vi "Init TCP.vi"(8 "error in (no error)":errorcluster, 11 "Vecto in":refnum<class "Vecto.lvclass">) -> (0 "error out":errorcluster, 3 "Vecto out":refnum<class "Vecto.lvclass">)   [LabVIEW 2020, in "Vecto.lvlib" / "Vecto.lvclass"]
uses:
  Vecto.lvclass
  Node Config/Node Config.lvclass
  TCPMessaging/TCPMessaging.lvclass
  VectoTCPConnectionHandler/VectoTCPConnectionHandler.lvclass
  proto/TcpClientHello/Data.ctl
  proto/TcpClientHello/TcpClientHello.lvlib
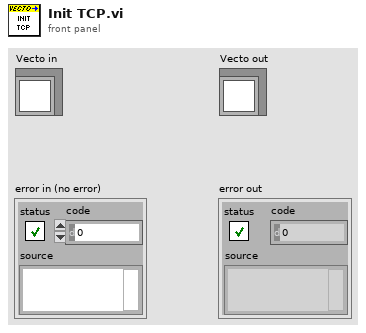
[diagram p1: front panel]
types:
  T1 = typedef "TcpClientHello.lvlib/Data.ctl" = cluster{"node_id":u32, "system":string, "cluster":string, "node_name":string, "app_version":string, "config_version":string}
  T2 = typedef "Vecto.lvlib/Node Config.lvclass/Node Info.ctl" = cluster{"System":string, "Cluster":string, "Name":string, "ID":u32}
  T3 = typedef "Vecto.lvlib/Node Config.lvclass/TCP Messaging Info.ctl" = cluster{"Address":string, "Port":u16, "Server (Client)":bool}
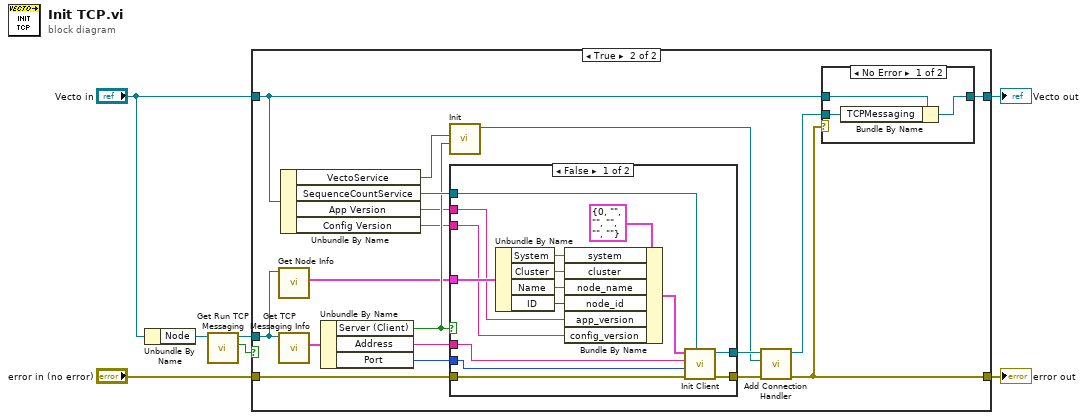
[diagram p0: block diagram]
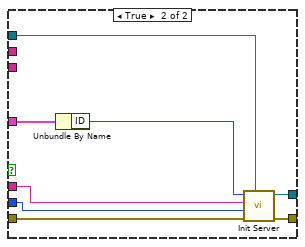
[diagram p3: hidden frame]
diagram:
  n1 = Unbundle By Name("Vecto in") -> ("Node"=w7:refnum<class "Node Config.lvclass">)
  n2 = call "Get Run TCP Messaging.vi"("Node Config in"=w7) -> ("Run TCP Messaging"=w6:bool, "Node Config out"=w4:refnum<class "Node Config.lvclass">)  [unwired: 8 in, 1 out]
  n3 = case shown="True" w6 {
    tunnel: "error in (no error)" -> [w8 w27]
    tunnel: w4 -> [_ w13]
    tunnel: "Vecto in" -> [w9 w22]
    tunnel: [w8 w17] -> w2
    tunnel: [w9 w21] -> w1
    frame False {
    }
    frame True {
      n4 = call "Get Node Info.vi"("Node Config in"=w13) -> ("Info"=w12:T2)  [unwired: 8 in, 2 out]
      n5 = call "Get TCP Messaging Info.vi"("Node Config in"=w13) -> ("TCP Messaging Info"=w26:T3)  [unwired: 8 in, 2 out]
      n6 = Unbundle By Name(w22) -> ("VectoService"=w19:refnum<class "VectoInfo.lvclass">, "SequenceCountService"=w23:refnum<class "SequenceCountService.lvclass">, "App Version"=w10:string, "Config Version"=w11:string)
      n7 = Unbundle By Name(w26) -> ("Server (Client)"=w18:bool, "Address"=w25:string, "Port"=w24:u16)
      n8 = call "Init.vi"("Server (Client)"=w18, "VectoInfo"=w19) -> ("VectoTCPConnectionHandler out"=w14:refnum<class "VectoTCPConnectionHandler.lvclass">)  [unwired: 8 in, 1 out]
      n9 = case shown="False" w18 {
        tunnel: w27 -> [w42 w50]
        tunnel: w25 -> [w32 w49]
        tunnel: w24 -> [w31 w48]
        tunnel: w23 -> [w39 w47]
        tunnel: [w40 w46] -> w16
        tunnel: [w41 w45] -> w20
        tunnel: w12 -> [w36 w44]
        tunnel: w11 -> [w30 _]
        tunnel: w10 -> [w29 _]
        frame False {
          n10 = Unbundle By Name(w36) -> ("System"=w35:string, "Cluster"=w34:string, "Name"=w33:string, "ID"=w28:u32)
          n11 = Bundle By Name(cluster=T1 {"node_id"=0, "system"="", "cluster"="", "node_name"="", "app_version"="", "config_version"=""} ("Client Info"), "system"=w35, "cluster"=w34, "node_name"=w33, "node_id"=w28, "app_version"=w29, "config_version"=w30) -> (w37:T1)
          n12 = call "Init Client.vi"("SequenceCountService"=w39, "error in (no error)"=w42, "Remote Port"=w31, "Remote Address"=w32, "Client Info"=w37) -> ("error out"=w41:errorcluster, "TCPMessaging out"=w40:refnum<class "TCPMessaging.lvclass">)  [unwired: 5 in]
        }
        frame True {
          n13 = Unbundle By Name(w44) -> ("ID"=w43:u32)
          n14 = call "Init Server.vi"("SequenceCountService"=w47, "error in (no error)"=w50, "Bind Port"=w48, "Bind Address"=w49, "Node ID"=w43) -> ("error out"=w45:errorcluster, "TCPMessaging out"=w46:refnum<class "TCPMessaging.lvclass">)  [unwired: 5 in]
        }
      }
      n15 = call "Add Connection Handler.vi"("error in (no error)"=w20, "TCPConnectionHandler"=w14, "TCPMessaging in"=w16) -> ("error out"=w17:errorcluster, "TCPMessaging out"=w15:refnum<class "TCPMessaging.lvclass">)  [unwired: 7 in]
      n16 = case shown="No Error" w17 {
        tunnel: w22 -> [w53 w54]
        tunnel: w15 -> [w52 _]
        tunnel: [w51 w54] -> w21
        frame No Error {
          n17 = Bundle By Name(cluster=w53, "TCPMessaging"=w52) -> (w51:refnum<class "Vecto.lvclass">)
        }
        frame Error {
        }
      }
    }
  }
  "error out" <- w2
  "Vecto out" <- w1
